vi "Find who is starting Module.vi"(7 "App Ref":refnum<vi>, 10 "Theme":bool=TRUE, 11 "Library in":refnum<vi>) -> ()   [LabVIEW 2019, in "Panther Dashboard.lvlib"]
uses:
  Panther Dashboard.lvlib
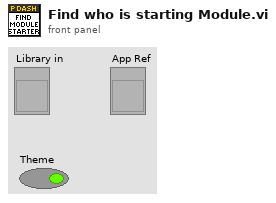
[diagram p1: front panel]
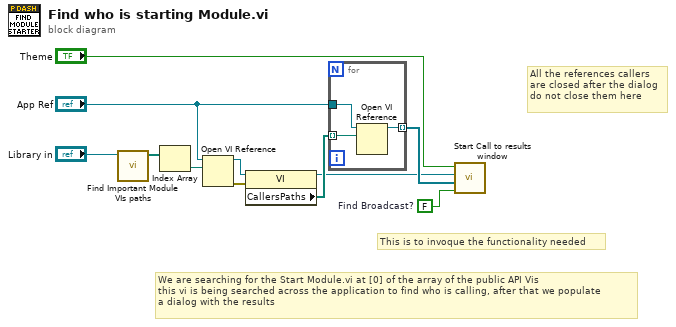
[diagram p0: block diagram]
diagram:
  w1 = FALSE  # Find Broadcast?
  # "All the references callers\nare closed after the dialog\ndo not close them here"
  # "This is to invoque the functionality needed"
  # "We are searching for the Start Module.vi at [0] of the array of the public API Vis\nthis vi is being searched across the application to find who is calling, after that we populate\na dialog with the results"
  n1 = call "Find Important Module VIs paths.vi"("Library in"="Library in") -> ("Public API VIs Paths"=w9:path[])  [unwired: 10 in]
  n2 = Index Array(array=w9) -> (element=w8:path)  [unwired: 1 in]
  n3 = Open VI Reference(application reference (local)="App Ref", vi path=w8) -> (vi reference=w7:refnum<vi>, error out=w11:errorcluster)  [unwired: 4 in]
  n4 = property class="VI"(reference=w7, error in=w11) -> (reference out=w3:refnum<vi>, "CallersPaths"=w5:path[])  [unwired: 1 out]
  n5 = for {
    tunnel: "App Ref" -> [w14]
    tunnel: w5 -> [w13] mode=indexing
    tunnel: [w12] -> w4 mode=indexing
    n6 = Open VI Reference(application reference (local)=w14, vi path=w13) -> (vi reference=w12:refnum<vi>)  [unwired: 4 in, 1 out]
  }
  n7 = call "Start Call to results window.vi"("Find Broadcast?"=w1, "Request VI Callers"=w4, "Event"=w3, "Theme"="Theme") -> ()  [unwired: 8 in]
